vi "niDTS BT LE Tx Test Initiate.vi"(0 "Dummy Test Handle In":T1, 11 "error in (no error)":errorcluster) -> (4 "Dummy Test Handle Out":T1, 15 "error out":errorcluster)   [LabVIEW 2014, in "niDTS BT.lvlib"]
uses:
  niDTS BT.lvlib
  Tx Test/Includes/niDTS BT Tx Test INC Handle.ctl
  Tx Test/Objects/BASE_class/niDTS BT Tx Test.lvclass
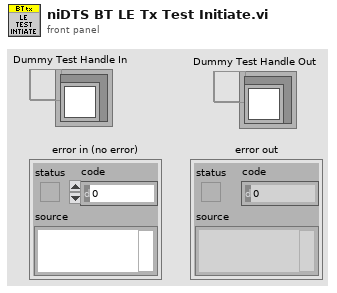
[diagram p1: front panel]
types:
  T1 = typedef "niDTS BT.lvlib/niDTS BT Tx Test INC Handle.ctl" = refnum<data-value>
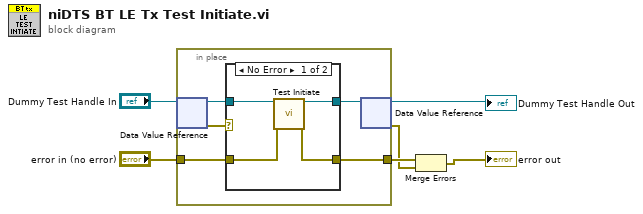
[diagram p0: block diagram]
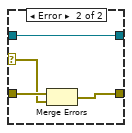
[diagram p2: hidden frame]
diagram:
  n1 = in-place {
    in-place-border: "error in (no error)" -> [w8]
    in-place-border: [w7] -> w3
    n2 = in-place-dvr #1("Dummy Test Handle In") -> (w10:refnum<class "niDTS BT Tx Test.lvclass">, w11:errorcluster)
    n3 = case shown="No Error" w11 {
      selector: w11 -> [_ w17]
      tunnel: w10 -> [w15 w19]
      tunnel: [w14 w19] -> w9
      tunnel: w8 -> [w13 w18]
      tunnel: [w12 w16] -> w7
      frame No Error {
        n4 = call-dynamic "Test Initiate.vi"("Template Tx Test in"=w15, "error in (no error)"=w13) -> ("Template Tx Test out"=w14:refnum<class "niDTS BT Tx Test.lvclass">, "error out"=w12:errorcluster)  [unwired: 12 in]
      }
      frame Error {
        n5 = Merge Errors(w18, w17) -> (w16:errorcluster)
      }
    }
    n6 = in-place-dvr #1(w9) -> (→"Dummy Test Handle Out":T1, w2:errorcluster)
  }
  n7 = Merge Errors(w3, w2) -> (→"error out":errorcluster)
